vi "Teleop-System-Globals.vi"() -> ()   [LabVIEW 2019]
panel:
  out "Joy0-POV":i32[](array[numeric])
  out "Joy0-Buttons":bool[](array[boolean])
  out "Joy0-Axes":dbl[](array[numeric])
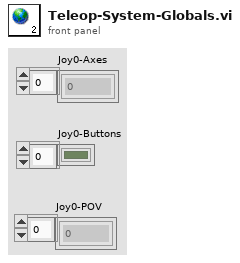
[diagram p1: front panel]
diagram:
